vi "CheckIfDirty.vi"(8 "error in":errorcluster, 9 "Saved Tree":T1[](array[typedef]), 11 "Tree Control":refnum<vi>) -> (0 "error out":errorcluster, 1 "Dirty Flag":bool, 2 "Current Tree":T1[](array[typedef]))   [LabVIEW 2010]
uses:
  ScriptStepTypeDef.ctl
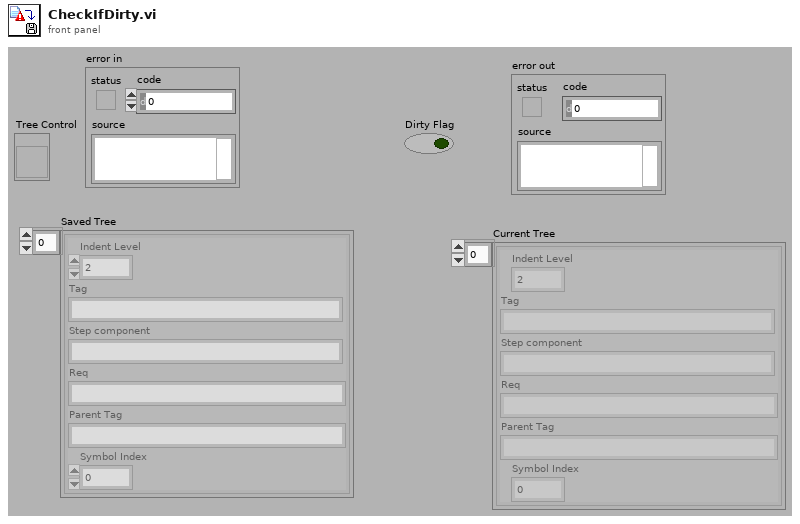
[diagram p1: front panel]
types:
  T1 = typedef "ScriptStepTypeDef.ctl" = cluster{"Indent Level":i32, "Tag":string, "Step component":string, "Req":string, "Parent Tag":string, "Symbol Index":i32}
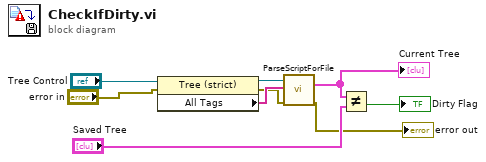
[diagram p0: block diagram]
diagram:
  n1 = property class="Tree (strict)"(reference="Tree Control", error in="error in") -> (reference out=w3:refnum<vi>, error out=w4:errorcluster, "All Tags"=w5:string[])
  n2 = call "ParseScriptForFile.vi"("Tree Ref in"=w3, "Script Array"=w5, "error in"=w4) -> ("Script Steps"=w6:T1[], "error out"=→"error out":errorcluster)  [unwired: 10 in, 1 out]
  "Current Tree" <- w6
  n3 = Not Equal?(x=w6, y="Saved Tree") -> (x != y?=→"Dirty Flag":bool)
